vi "savetimestamps.vi"(1 "timestamp":timestamp, 2 "filename prefix in":string, 3 "data dir in":path=path "C:/Users/Labmember/Desktop/Data/temp" caption="data dir.") -> ()   [LabVIEW 2015]
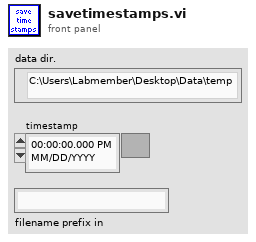
[diagram p1: front panel]
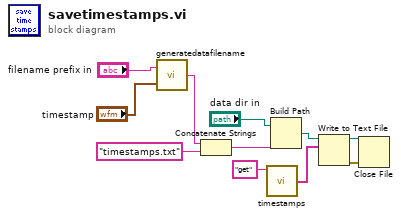
[diagram p0: block diagram]
diagram:
  n1 = call "generatedatafilename.vi"("timestamp"="timestamp", "filename prefix in"="filename prefix in") -> ("full-filename"=w1:string)
  n2 = Concatenate Strings(w1, "timestamps.txt" ("string")) -> (w9:string)
  n3 = call "timestamps.vi"("command"="get") -> ("timestamps out"=w4:string[])  [unwired: 3 in]
  n4 = Build Path(base path="data dir in", name or relative path=w9) -> (appended path=w6:path)
  n5 = Write to Text File(file (use dialog)=w6, text=w4) -> (refnum out=w8:refnum<file>, error out=w7:errorcluster)  [unwired: 2 in, 1 out]
  n6 = Close File(refnum=w8, error in=w7) -> ()  [unwired: 2 out]
